vi "Clear Configuration.vi"(8 "error in (no error)":errorcluster, 11 "Item Ref in":T1 format="%.0x") -> (0 "error out":errorcluster)   [LabVIEW 2015, in "DCM System Explorer.lvlib"]
uses:
  DCM System Explorer.lvlib
  <vilib>/NI Veristand/Custom Device API/Custom Device Item Ref.ctl
  <vilib>/NI VeriStand/Custom Device API/Custom Device API.lvlib
  <vilib>/NI Veristand/Custom Device Tools/Custom Device Utility Library/Custom Device Utility Library.lvlib
  <vilib>/NI Veristand/Custom Device Tools/Custom Device Utility Library/NI VeriStand - Search for All Items by GUID.vi
  Shared/DCM Constants and GUIDs.vi
  DCM Shared.lvlib
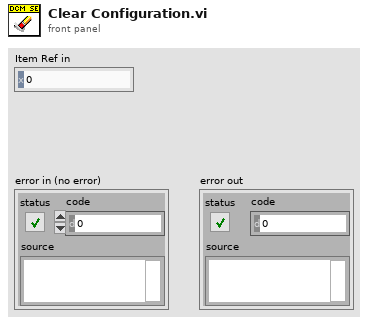
[diagram p1: front panel]
types:
  T1 = typedef "Custom Device API.lvlib/Custom Device Item Ref.ctl" = u64
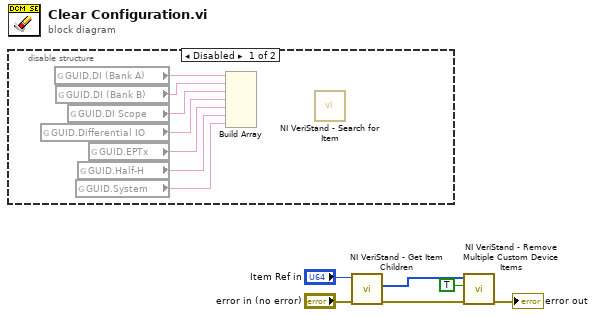
[diagram p0: block diagram]
diagram:
  n1 = disable-structure shown="Disabled" {
    frame Disabled {
      n2 = global read "DCM Constants and GUIDs.vi" "GUID.Differential IO"() -> (w10:string)
      n3 = global read "DCM Constants and GUIDs.vi" "GUID.DI (Bank A)"() -> (w13:string)
      n4 = global read "DCM Constants and GUIDs.vi" "GUID.DI (Bank B)"() -> (w12:string)
      n5 = global read "DCM Constants and GUIDs.vi" "GUID.DI Scope"() -> (w11:string)
      n6 = global read "DCM Constants and GUIDs.vi" "GUID.System"() -> (w7:string)
      n7 = global read "DCM Constants and GUIDs.vi" "GUID.Half-H"() -> (w8:string)
      n8 = global read "DCM Constants and GUIDs.vi" "GUID.EPTx"() -> (w9:string)
      n9 = Build Array(w13, w12, w11, w10, w9, w8, w7) -> ()  [unwired: 1 out]
      n10 = call-poly <vilib>:"NI VeriStand - Search for Item.vi"() -> ()  [unwired: 8 in, 4 out]
    }
    frame Enabled {
    }
  }
  n11 = call <vilib>:"NI VeriStand - Get Item Children.vi"("error in (no error)"="error in (no error)", "Item Ref in"="Item Ref in") -> ("error out"=w2:errorcluster, "Child Refs"=w1:T1[])  [unwired: 6 in, 2 out]
  n12 = call <vilib>:"NI VeriStand - Remove Multiple Custom Device Items.vi"("error in (no error)"=w2, "Force Delete (F)"=TRUE, "Item Refs in"=w1) -> ("error out"=→"error out":errorcluster)  [unwired: 7 in, 1 out]
